vi "WrongCRCPacket.vi"() -> (3 "string":string)   [LabVIEW 2018]
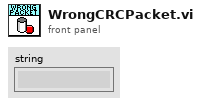
[diagram p1: front panel]
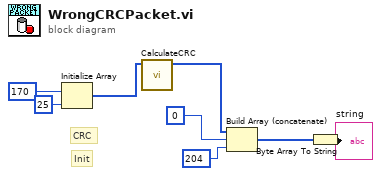
[diagram p0: block diagram]
diagram:
  # "Init"
  # "CRC"
  n1 = Initialize Array(u8 170, 25 ("dimension size")) -> (w2:u8[])
  n2 = call "CalculateCRC.vi"("data in"=w2) -> ("data out"=w1:u8[])  [unwired: 9 in, 1 out]
  n3 = Build Array (concatenate)(w1, u8 0, u8 204) -> (w4:u8[])
  n4 = Byte Array To String(unsigned byte array=w4) -> (string=→"string":string)
